vi "TO_counts.vi"(8 "error in (no error)":errorcluster, 11 "State Machine in":refnum<class "State Machine.lvclass">) -> (0 "error out":errorcluster, 2 "timer zero":bool, 3 "State Machine out":refnum<class "State Machine.lvclass">)   [LabVIEW 2018, in "State Machine.lvclass"]
uses:
  State Machine.lvclass
  State Machine.lvclass/State Machine.ctl
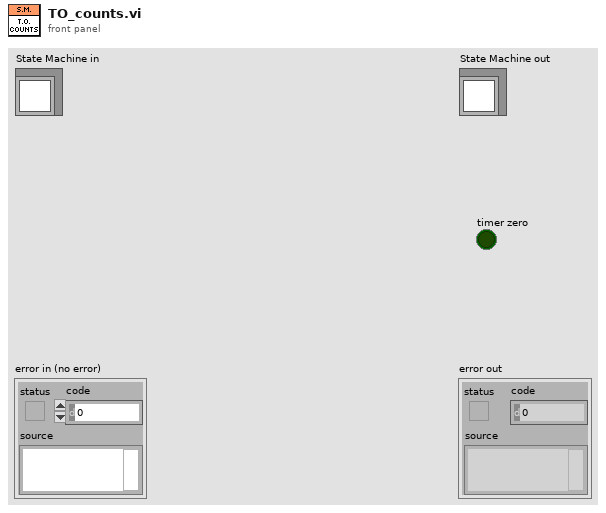
[diagram p1: front panel]
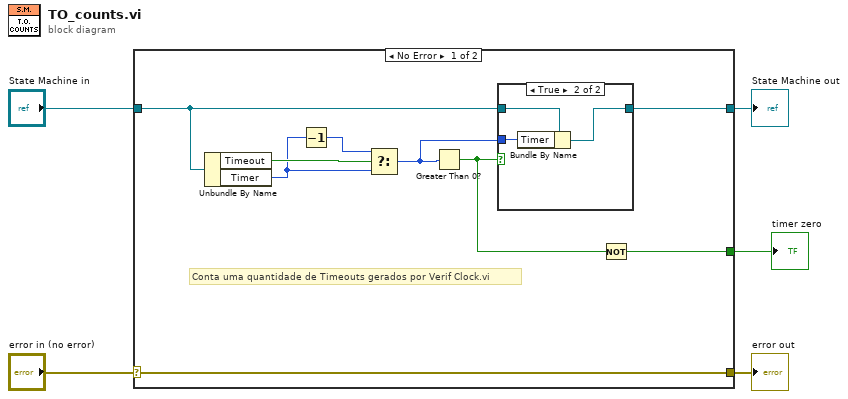
[diagram p0: block diagram]
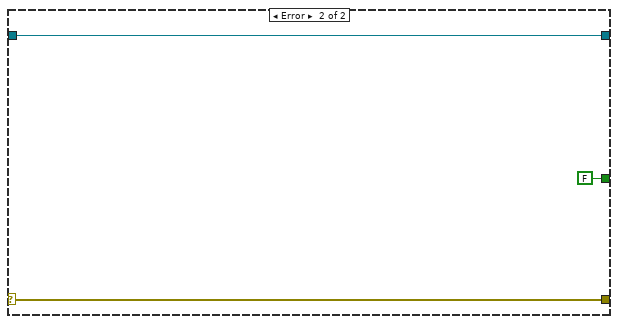
[diagram p3: hidden frame]
diagram:
  n1 = case shown="No Error" "error in (no error)" {
    selector: "error in (no error)" -> [w14 w21]
    tunnel: [w14 w21] -> w4
    tunnel: [w9 w20] -> w2
    tunnel: "State Machine in" -> [w10 w20]
    tunnel: [w6 FALSE] -> w1
    frame No Error {
      # "Conta uma quantidade de Timeouts gerados por Verif Clock.vi"
      n2 = Unbundle By Name(w10) -> ("Timeout"=w13:bool, "Timer"=w12:u32)
      n3 = Decrement(x=w12) -> (x-1=w11:u32)
      n4 = Select(t=w11, s=w13, f=w12) -> (s? t:f=w8:u32)
      n5 = Greater Than 0?(x=w8) -> (x > 0?=w7:bool)
      n6 = case shown="True" w7 {
        tunnel: w10 -> [w15 w18]
        tunnel: [w15 w17] -> w9
        tunnel: w8 -> [_ w16]
        frame False {
        }
        frame True {
          n7 = Bundle By Name(cluster=w18, "Timer"=w16) -> (w17:refnum<class "State Machine.lvclass">)
        }
      }
      n8 = Not(x=w7) -> (.not. x?=w6:bool)
    }
    frame Error {
    }
  }
  "error out" <- w4
  "State Machine out" <- w2
  "timer zero" <- w1
